vi "Startup.vi"(7 "App":refnum<class>, 8 "error in (no error)":errorcluster, 9 "Base LogFolder":path, 10 "Config":refnum<class>, 11 "DbgTimers in":refnum<class "DbgTimers.lvclass">) -> (0 "error out":errorcluster, 3 "DbgTimers out":refnum<class "DbgTimers.lvclass">)   [LabVIEW 2017, in "DbgTimers.lvclass"]
doc: "Developed by Kevin Thompson\nkevin@thompsonengineering.net\n\nCopyright 2018-2020\nThompson Engineering, LLC"
uses:
  DbgTimers.lvclass
  DataTypes/Dependency--cluster.ctl
  DataTypes/Settings--cluster.ctl
  Ichor_Common/DataTypes/TD GetSet ActionSelect--enum.ctl
  DbgTimers.lvclass/DbgTimers.ctl
  Accessors/Set Dependency.vi
  Accessors/Set Enable msTick Logging.vi
  Accessors/Set Settings.vi
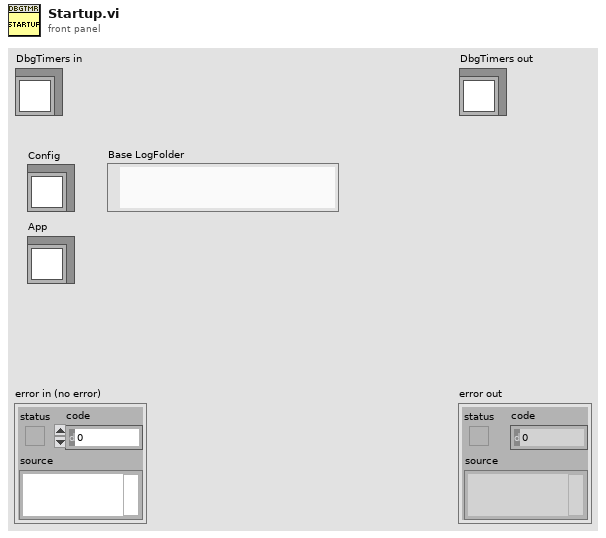
[diagram p1: front panel]
types:
  T1 = typedef "TD GetSet ActionSelect--enum.ctl" = enum16{"Init", "Get", "Set"}
  T2 = typedef "DbgTimers.lvclass/Settings--cluster.ctl" = cluster{"Simulation":bool, "DbgTimer LogFolder":path}
  T3 = typedef "DbgTimers.lvclass/Dependency--cluster.ctl" = cluster{"Config":refnum<class>, "ClassRef":refnum<class>}
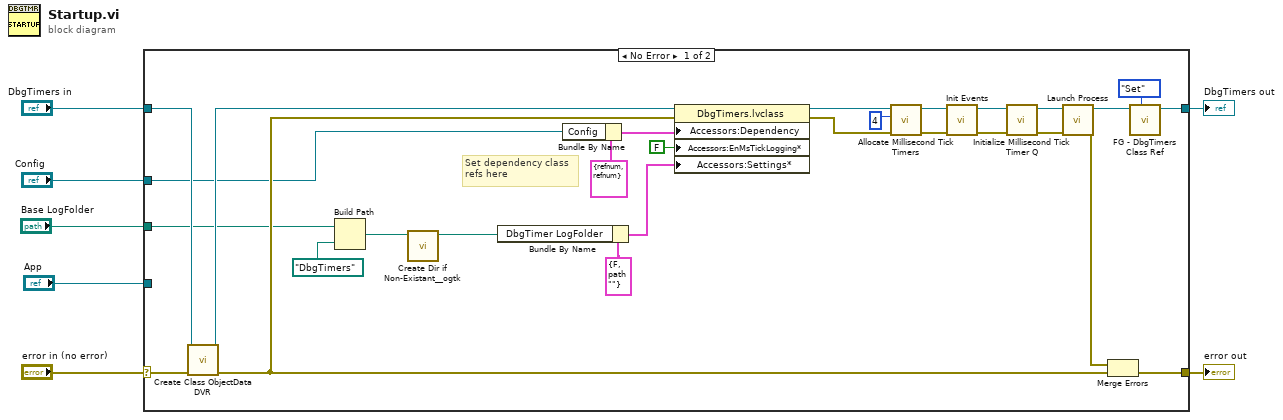
[diagram p0: block diagram]
diagram:
  n1 = case shown="No Error" "error in (no error)" {
    selector: "error in (no error)" -> [w35 w37]
    tunnel: [w32 w37] -> w6
    tunnel: [w14 w36] -> w4
    tunnel: "DbgTimers in" -> [w34 w36]
    tunnel: "Config" -> [w28 _]
    tunnel: "App" -> [_ _]
    tunnel: "Base LogFolder" -> [w22 _]
    frame No Error {
      # "Set dependency class\nrefs here"
      n2 = call "Create Class ObjectData DVR.vi"("error in (no error)"=w35, "DbgTimers in"=w34) -> ("error out"=w30:errorcluster, "DbgTimers out"=w33:refnum<class "DbgTimers.lvclass">)  [unwired: 8 in]
      n3 = Build Path(base path=w22, name or relative path=path "DbgTimers") -> (appended path=w23:path)
      n4 = call <userlib>:"Create Dir if Non-Existant__ogtk.vi"("Directory Path"=w23) -> ("dup Directory Path"=w16:path)  [unwired: 8 in, 2 out]
      n5 = Bundle By Name(cluster=T2 {"Simulation"=FALSE, "DbgTimer LogFolder"=path ""} ("Settings*"), "DbgTimer LogFolder"=w16) -> (w24:T2)
      n6 = Bundle By Name(cluster=T3 {"Config"=refnum, "ClassRef"=refnum} ("Dependency"), "Config"=w28) -> (w27:T3)
      n7 = property class="DbgTimers.lvclass"(reference=w33, error in=w30, "Accessors:Dependency"=w27, "Accessors:EnMsTickLogging*"=FALSE ("EnMsTickLogging*"), "Accessors:Settings*"=w24) -> (reference out=w12:refnum<class "DbgTimers.lvclass">, error out=w10:errorcluster)
      n8 = call "Allocate Millisecond Tick Timers.vi"("error in (no error)"=w10, "QtyTimers"=4, "DbgTimers in"=w12) -> ("error out"=w9:errorcluster, "DbgTimers out"=w11:refnum<class "DbgTimers.lvclass">)  [unwired: 7 in]
      n9 = call "Init Events.vi"("error in (no error)"=w9, "DbgTimers in"=w11) -> ("error out"=w17:errorcluster, "DbgTimers out"=w20:refnum<class "DbgTimers.lvclass">)  [unwired: 8 in]
      n10 = call "Initialize Millisecond Tick Timer Q.vi"("error in (no error)"=w17, "DbgTimers in"=w20) -> ("error out"=w18:errorcluster, "DbgTimers out"=w19:refnum<class "DbgTimers.lvclass">)  [unwired: 8 in]
      n11 = call "Launch Process.vi"("error in (no error)"=w18, "DbgTimers in"=w19) -> ("error out"=w31:errorcluster, "DbgTimers out"=w15:refnum<class "DbgTimers.lvclass">)  [unwired: 6 in, 2 out]
      n12 = Merge Errors(w31, w30) -> (w32:errorcluster)
      n13 = call "FG - DbgTimers Class Ref.vi"("DbgTimers in"=w15, "action (Get)"=TD_GetSet_ActionSelect--enum."Set") -> ("DbgTimers out"=w14:refnum<class "DbgTimers.lvclass">)  [unwired: 7 in, 1 out]
    }
    frame Error {
    }
  }
  "error out" <- w6
  "DbgTimers out" <- w4
